vi "Core Write DAQ DVR FIFO.vi"(6 "FIFO Timestamps":T1, 8 "error in (no error)":errorcluster, 9 "Timeout (ms)":i32=100, 10 "Data In":refnum<data-value>[](array[refnum]), 11 "CIFTag in":refnum<class "CIF_NIChn_Fifo_DAQ.lvclass">) -> (0 "error out":errorcluster, 1 "timed out?":bool, 2 "Data Out":refnum<data-value>[](array[refnum]), 3 "CIFTag out":refnum<class "CIF_NIChn_Fifo_DAQ.lvclass">)   [LabVIEW 2021, in "CIF_NIChn_Fifo_DAQ.lvclass"]
uses:
  CIF_NIChn_Fifo_DAQ.lvclass
  D:/dev/CIF-LVCore/src/Channels/CIF_NIChn/NIChn/CIF_NIChn.lvclass
  ChannelCommon/typedef/TimeStamps.ctl
  ChannelCommon/typedef/Datatype Waveform.ctl
  CIF_NIChn_Fifo_DAQ.lvclass/CIF_NIChn_Fifo_DAQ.ctl
  ChannelCommon/CIFFIFO/CIFfifo.lvclass/CIFfifo.ctl
  NIChn/CIF_NIChn.lvclass/CIF_NIChn.ctl
  ChannelCommon/CIFFIFO/Accessors/Read Length.vi
  CIFCore/Common/Utilities/Append Error Location.vi
  <vilib>/CIFChannels/SubVIs/Get dll Path.vi
  ChannelCommon/CIFFIFO/Utilities/Update Header.vi
  ChannelCommon/CIFFIFO/Flatten/DVR Flatten.vi
  ChannelCommon/CIFFIFO/Accessors/Write T0.vi
  ChannelCommon/CIFFIFO/Accessors/Write T_Out.vi
  ChannelCommon/CIFFIFO/Accessors/Write ClockID.vi
  ChannelCommon/Utilities/Flatten Header.vi
  ChannelCommon/CIFFIFO/Flatten/DVR Flatten.vi/6fdbece9-bad6-4a8e-9bf7-fe1528478dd6.vi
  ChannelCommon/CIFFIFO/Accessors/Write Payload Length.vi
  ChannelCommon/CIFFIFO/Accessors/Read Header.vi
  CIFCore/Common/Utilities/Add Error.vi
  ChannelCommon/CIFFIFO/Flatten/DVR Flatten.vi/6fdbece9-bad6-4a8e-9bf7-fe1528478dd6.vi/c28b0ead-42ad-4072-80a2-aca7f2bd7ce3.vi
  ChannelCommon/Utilities/Update Time.vi
  NIChn/CIF_NIChn.lvclass
  <vilib>/CIFChannels/CIFChannelCore.lvlib
  ChannelCommon/CIFFIFO/CIFfifo.lvclass
  ChannelCommon/ChannelCommon.lvlib
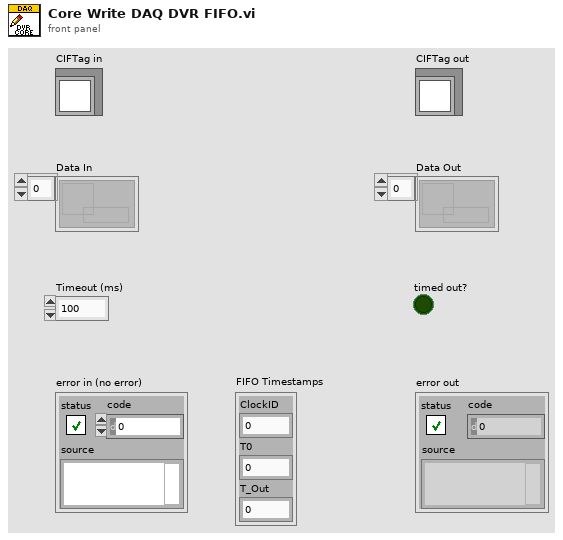
[diagram p1: front panel]
types:
  T1 = typedef "ChannelCommon.lvlib/TimeStamps.ctl" = cluster{"ClockID":u8, "T0":u64, "T_Out":u64}
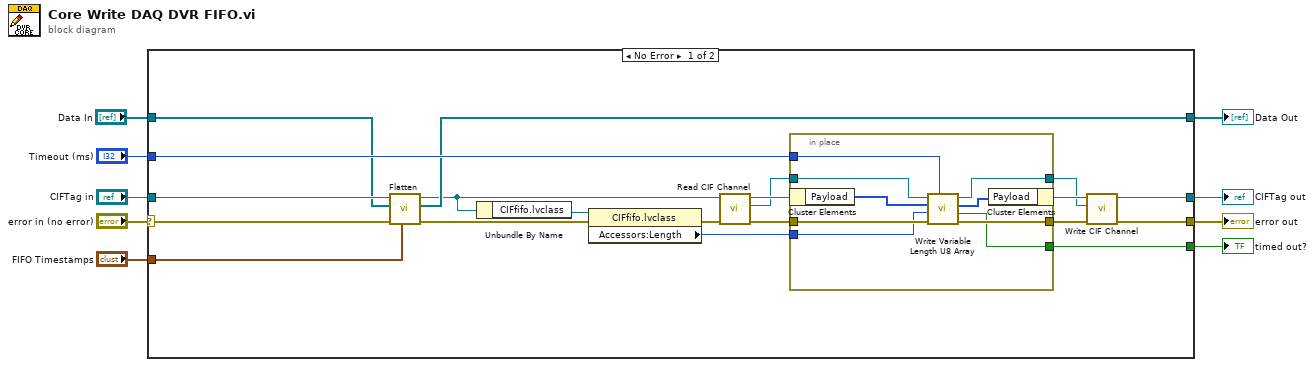
[diagram p0: block diagram]
diagram:
  n1 = case shown="No Error" "error in (no error)" {
    selector: "error in (no error)" -> [w24 w41]
    tunnel: [w26 w41] -> w8
    tunnel: [w28 w40] -> w6
    tunnel: "CIFTag in" -> [w25 w40]
    tunnel: [w29 _] -> w5
    tunnel: "Timeout (ms)" -> [w27 _]
    tunnel: [w23 w39] -> w1
    tunnel: "Data In" -> [w22 w39]
    tunnel: "FIFO Timestamps" -> [w21 _]
    frame No Error {
      n2 = call "Flatten.vi"("FIFO Timestamps"=w21, "error in (no error)"=w24, "Data In"=w22, "CIFTag in"=w25) -> ("error out"=w11:errorcluster, "Data Out"=w23:refnum<data-value>[], "CIFTag out"=w12:refnum<class "CIF_NIChn_Fifo_DAQ.lvclass">)  [unwired: 5 in]
      n3 = Unbundle By Name(w12) -> ("CIFfifo.lvclass"=w14:refnum<class "CIFfifo.lvclass">)
      n4 = property class="CIFfifo.lvclass"(reference=w14, error in=w11) -> (error out=w13:errorcluster, "Accessors:Length"=w10:u64)  [unwired: 1 out]
      n5 = call "Read CIF Channel.vi"("error in (no error)"=w13, "CIFTag in"=w12) -> ("error out"=w19:errorcluster, "CIF Channel"=w16:refnum<k21>, "CIFTag out"=w20:refnum<class "CIF_NIChn_Fifo_DAQ.lvclass">)  [unwired: 7 in]
      n6 = in-place {
        in-place-border: w19 -> [w38]
        in-place-border: [w37] -> w17
        in-place-border: [w36] -> w29
        in-place-border: w16 -> [w35]
        in-place-border: [w34] -> w15
        in-place-border: w27 -> [w33]
        in-place-border: w10 -> [w31]
        n7 = in-place-cluster #1(w20) -> ("Payload"=w32:u8[])
        n8 = call <vilib>:"Write Variable Length U8 Array.vi"("Timeout (ms)"=w33, "error in"=w38, "numElements"=w31, "U8 Array in"=w32, "CIF Channel in"=w35) -> ("error out"=w37:errorcluster, "Timed out?"=w36:bool, "U8 Array out"=w30:u8[], "CIF Channel out"=w34:refnum<k21>)  [unwired: 3 in]
        n9 = in-place-cluster #1("Payload"=w30) -> (w18:refnum<class "CIF_NIChn_Fifo_DAQ.lvclass">)
      }
      n10 = call "Write CIF Channel.vi"("error in (no error)"=w17, "CIF Channel"=w15, "CIFTag in"=w18) -> ("error out"=w26:errorcluster, "CIFTag out"=w28:refnum<class "CIF_NIChn_Fifo_DAQ.lvclass">)  [unwired: 7 in]
    }
    frame Error {
    }
  }
  "error out" <- w8
  "CIFTag out" <- w6
  "timed out?" <- w5
  "Data Out" <- w1
